vi "ServiceTrigger.Compile.vi"(8 "error in (no error)":errorcluster, 10 "Settings":T3[](array[typedef]) {"Signal.Cmd.Refs"."Signal Refs" format="%.0x"; "Signal.Cmd.Info"."Signals"."Byte Order" items=["Little Endian", "Big Endian"]; "Signal.Cmd.Info"."Signals"."Data Type" items=["Signed", "Unsigned", "IEEE Float"]; "Settings.Refs"."Signal Refs" format="%.0x"; "Signal.Resp.Refs"."Signal Refs" format="%.0x"; "Signal.Resp.Info"."Signals"."Byte Order" items=["Little Endian", "Big Endian"]; "Signal.Resp.Info"."Signals"."Data Type" items=["Signed", "Unsigned", "IEEE Float"]; "Trigger.Refs"."Signal Refs" format="%.0x"; "Status.Refs"."Signal Refs" format="%.0x"}) -> (0 "error out":errorcluster, 2 "Refs":T2(array[cluster]) {"VS Refs" format="%.0x"}, 3 "Trigger Lookup":variant)   [LabVIEW 2019, in "Diagnostics Addon System Explorer.lvlib"]
uses:
  Diagnostics Addon System Explorer.lvlib
  Types/Service.Export.ctl
  Types/Frame.Ref.ctl
  Shared/Types/Type.ctl
  <vilib>/NI VeriStand/Custom Device API/Custom Device Item Ref.ctl
  Shared/Types/Frame.Compile.ctl
  Shared/Types/Signal.ctl
  Shared/Types/Trigger.Settings.ctl
  Shared/SubVIs/Constants.vi
  <vilib>/NI VeriStand/Custom Device API/Custom Device API.lvlib
  Shared/Diagnostics Addon Shared.lvlib
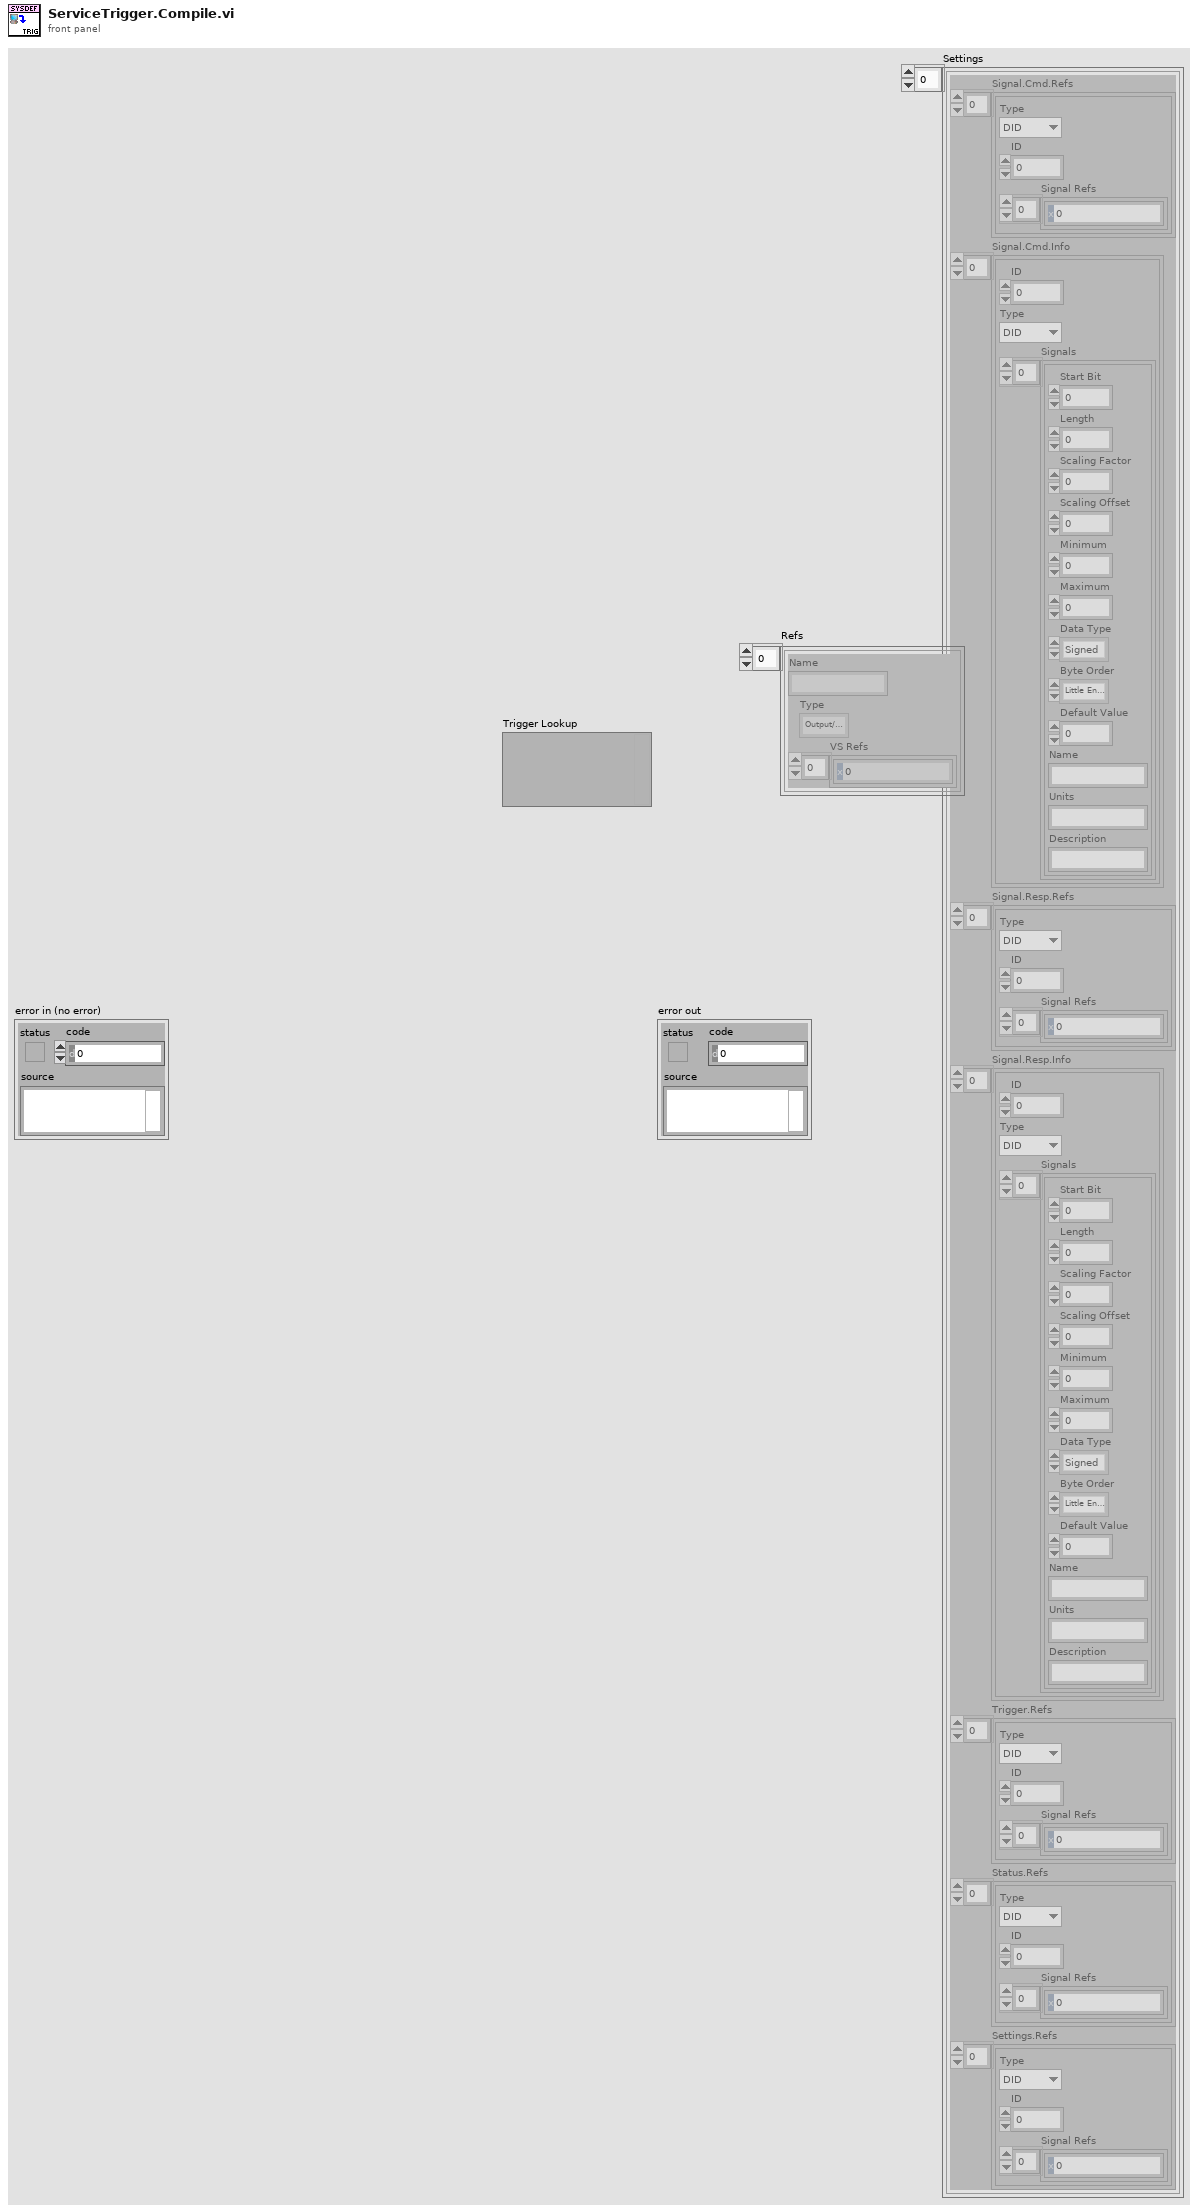
[diagram p1: front panel]
types:
  T1 = typedef "Custom Device API.lvlib/Custom Device Item Ref.ctl" = u64
  T2 = cluster{"Name":string, "Type":enum16{"Output/Write", "Input/Read", "Input/ReadWrite"}, "VS Refs":T1[]}[]
  T3 = typedef "Diagnostics Addon System Explorer.lvlib/Service.Export.ctl" = cluster{"Signal.Cmd.Refs":T4[], "Signal.Cmd.Info":T6[], "Signal.Resp.Refs":T4[], "Signal.Resp.Info":T6[], "Trigger.Refs":T4[], "Status.Refs":T4[], "Settings.Refs":T4[]}
  T4 = typedef "Diagnostics Addon System Explorer.lvlib/Frame.Ref.ctl" = cluster{"Type":T5, "ID":u32, "Signal Refs":T1[]}
  T5 = typedef "Diagnostics Addon Shared.lvlib/Type.ctl" = enum16{"DID", "CDID", "PID", "CPID", "Read Memory", "Write Memory", "DTC Control", "IO Cmd", "IO Resp", "Routine Start Cmd", "Routine Start Resp", "Routine Request Cmd", "Routine Request Resp", "Routine Stop Cmd", "Routine Stop Resp", "UserDefined Cmd", "UserDefined Rsp"}
  T6 = typedef "Diagnostics Addon Shared.lvlib/Frame.Compile.ctl" = cluster{"ID":u32, "Type":T5, "Signals":T7[]}
  T7 = typedef "Diagnostics Addon Shared.lvlib/Signal.ctl" = cluster{"Start Bit":u32, "Length":u32, "Scaling Factor":dbl, "Scaling Offset":dbl, "Minimum":dbl, "Maximum":dbl, "Data Type":u32, "Byte Order":u32, "Default Value":dbl, "Name":string, "Units":string, "Description":string}
  T8 = enum16{"Output/Write", "Input/Read", "Input/ReadWrite"}
  T9 = cluster{"Name":string, "Type":enum16{"Output/Write", "Input/Read", "Input/ReadWrite"}, "VS Refs":T1[]}
  T10 = typedef "Diagnostics Addon Shared.lvlib/Trigger.Settings.ctl" = cluster{"Type":T5, "ID":u32, "Settings?":bool, "Index":i32, "Length":i32}
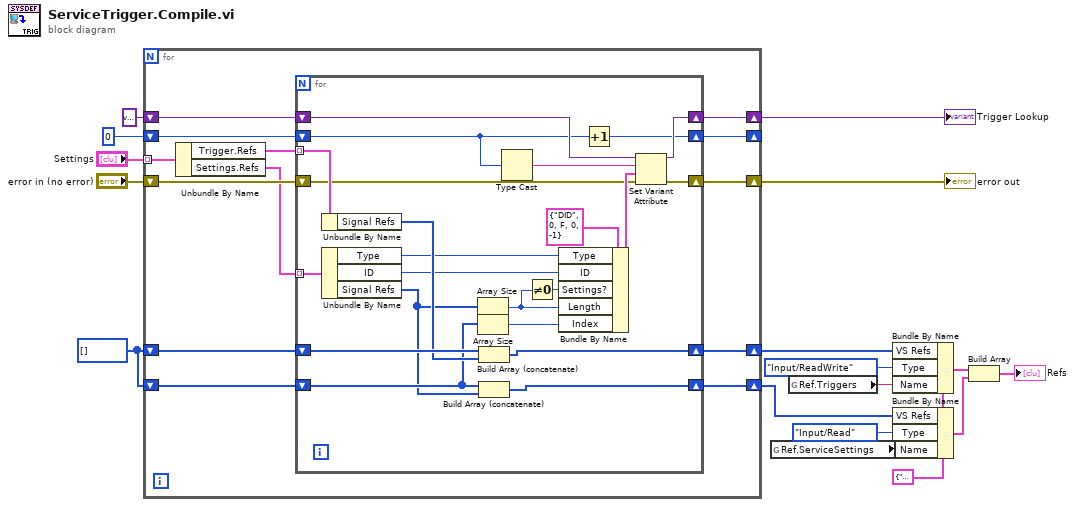
[diagram p0: block diagram]
diagram:
  w3 = T9 {"Name"="", "Type"=enum."Output/Write", "VS Refs"=[]} ("Group")
  w9 = T1[] []
  n1 = for {
    shift-right: [w25] -> w12
    shift-left: "error in (no error)" -> [w30]
    shift-right: [w29] -> w16
    shift-left: variant ("Lookup In") -> [w27]
    shift-right: [w26] -> w13
    shift-left: w9 -> [w28]
    tunnel: "Settings" -> [w24] mode=indexing
    shift-right: [w21] -> w6
    shift-left: w9 -> [w22]
    shift-right: [w19] -> _
    shift-left: u32 0 -> [w20]
    n2 = Unbundle By Name(w24) -> ("Trigger.Refs"=w23:T4[], "Settings.Refs"=w18:T4[])
    n3 = for {
      tunnel: w23 -> [w47] mode=indexing
      shift-right: [w48] -> w29
      shift-left: w27 -> [w51]
      shift-right: [w50] -> w25
      shift-left: w30 -> [w45]
      shift-right: [w44] -> w26
      shift-left: w28 -> [w46]
      shift-right: [w42] -> w21
      shift-left: w22 -> [w41]
      shift-right: [w38] -> w19
      shift-left: w20 -> [w39]
      tunnel: w18 -> [w32] mode=indexing
      n4 = Unbundle By Name(w47) -> ("Signal Refs"=w43:T1[])
      n5 = Unbundle By Name(w32) -> ("Type"=w34:T5, "ID"=w33:u32, "Signal Refs"=w37:T1[])
      n6 = Array Size(array=w37) -> (size(s)=w35:i32)
      n7 = Array Size(array=w41) -> (size(s)=w31:i32)
      n8 = Build Array (concatenate)(w46, w43) -> (w44:T1[])
      n9 = Build Array (concatenate)(w41, w37) -> (w42:T1[])
      n10 = Type Cast(x=w39) -> (*(type *) &x=w49:string)  [unwired: 1 in]
      n11 = Not Equal To 0?(x=w35) -> (x != 0?=w36:bool)
      n12 = Bundle By Name(cluster=T10 {"Type"=enum."DID", "ID"=0, "Settings?"=FALSE, "Index"=0, "Length"=-1} ("Cluster"), "Type"=w34, "ID"=w33, "Settings?"=w36, "Length"=w35, "Index"=w31) -> (w52:T10)
      n13 = Increment(x=w39) -> (x+1=w38:u32)
      n14 = Set Variant Attribute(Variant=w51, name=w49, value=w52, error in=w45) -> (Variant out=w48:variant, error out=w50:errorcluster)  [unwired: 1 out]
    }
  }
  "error out" <- w12
  "Trigger Lookup" <- w16
  n15 = global read "Constants.vi" "Ref.ServiceSettings"() -> (w7:string)
  n16 = global read "Constants.vi" "Ref.Triggers"() -> (w15:string)
  n17 = Bundle By Name(cluster=w3, "VS Refs"=w13, "Type"=T8."Input/ReadWrite", "Name"=w15) -> (w5:T9)
  n18 = Bundle By Name(cluster=w3, "VS Refs"=w6, "Type"=T8."Input/Read", "Name"=w7) -> (w4:T9)
  n19 = Build Array(w5, w4) -> (→"Refs":T2)
